vi "ATF-DO References FGV.vi"(7 "State":enum16{"Init", "Read", "Write"}(ring), 8 "error in":errorcluster, 11 "DO ref in":refnum<vi>[](array[refnum])) -> (0 "error out":errorcluster, 3 "DO ref out":refnum<vi>[](array[refnum]))   [LabVIEW 2022 SP3]
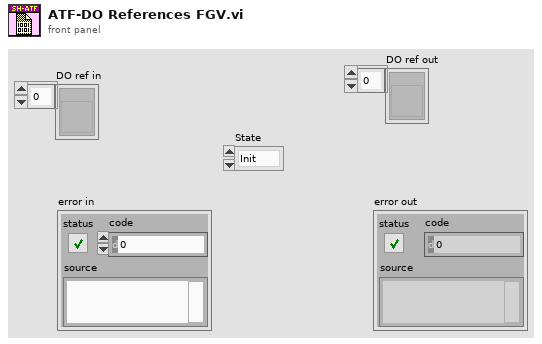
[diagram p1: front panel]
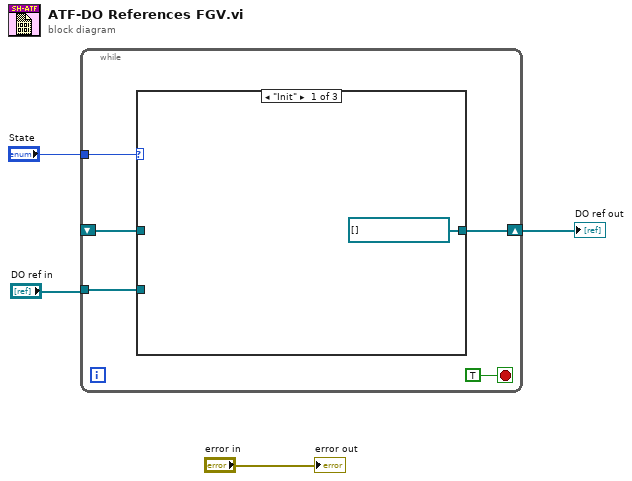
[diagram p0: block diagram]
diagram:
  n1 = while {
    shift-right: [w8] -> w2
    shift-left: _ -> [w9]
    tunnel: "DO ref in" -> [w7]
    tunnel: "State" -> [w5]
    stop <- TRUE stop-if-true
    n2 = case shown="\"Init\"" w5 {
      tunnel: w9 -> [_ w11 _]
      tunnel: [refnum<vi>[] [] ("appended array") w11 w12] -> w8
      tunnel: w7 -> [_ _ w12]
      frame "Init" {
      }
      frame "Read", Default {
      }
      frame "Write" {
      }
    }
  }
  "DO ref out" <- w2
  "error out" <- "error in"
